vi "GetImageDimensions.vi"(3 "2 nd Axis":u16, 4 "1st Axis":u16, 5 "Images Size (pixel)":cluster{u32, u32, u32}) -> (0 "planes":u32, 1 "lines":u32, 2 "columns":u32)   [LabVIEW 2009]
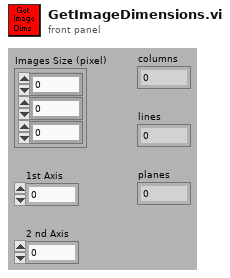
[diagram p1: front panel]
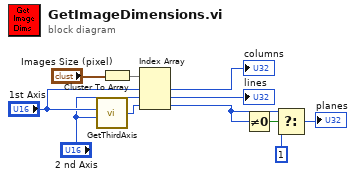
[diagram p0: block diagram]
diagram:
  n1 = call "GetThirdAxis.vi"("1st Axis"="2 nd Axis", "2nd Axis"="1st Axis") -> ("3rd Axis"=w7:i32)  [unwired: 2 in]
  n2 = Cluster To Array(cluster="Images Size (pixel)") -> (array=w6:u32[])
  n3 = Index Array(array=w6, index #1="1st Axis", index #2="2 nd Axis", index #3=w7) -> (element #1=→"columns":u32, element #2=→"lines":u32, element #3=w1:u32)
  n4 = Not Equal To 0?(x=w1) -> (x != 0?=w4:bool)
  n5 = Select(t=w1, s=w4, f=u32 1) -> (s? t:f=→"planes":u32)
